vi "Write outer terminal.vi"(5 "outer terminal":refnum<class "Terminal.lvclass">, 9 "Tunnel in":refnum<class "Tunnel.lvclass">) -> (3 "Tunnel out":refnum<class "Tunnel.lvclass">)   [LabVIEW 2014, in "Tunnel.lvclass"]
uses:
  Tunnel.lvclass
  Terminal/Terminal.lvclass
  Tunnel.lvclass/Tunnel.ctl
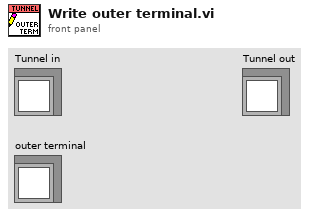
[diagram p1: front panel]
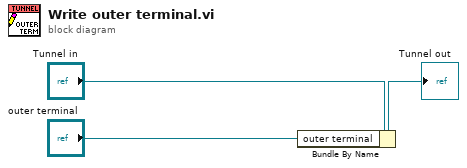
[diagram p0: block diagram]
diagram:
  n1 = Bundle By Name(cluster="Tunnel in", "outer terminal"="outer terminal") -> (→"Tunnel out":refnum<class "Tunnel.lvclass">)
